vi "查找匹配累积剂量.vi"(8 "探头名称":string, 11 "累积剂量":T2(array[cluster])) -> (0 "匹配？":bool, 2 "匹配索引":i32, 3 "匹配的累积剂量":T1)   [LabVIEW 2017]
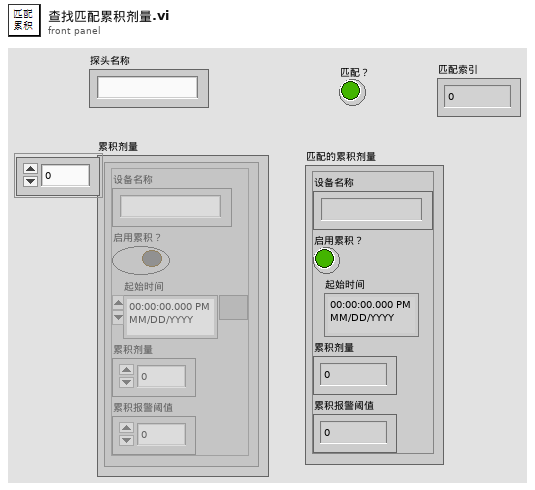
[diagram p1: front panel]
types:
  T1 = cluster{"设备名称":string, "启用累积？":bool, "起始时间":timestamp, "累积剂量":dbl, "累积报警阈值":dbl}
  T2 = cluster{"设备名称":string, "启用累积？":bool, "起始时间":timestamp, "累积剂量":dbl, "累积报警阈值":dbl}[]
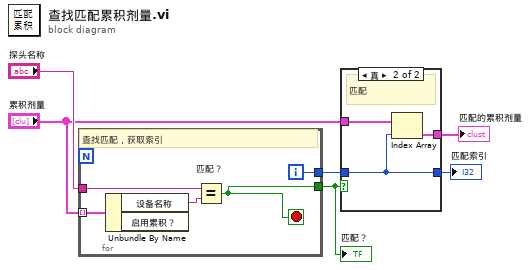
[diagram p0: block diagram]
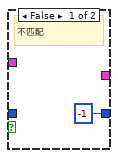
[diagram p2: hidden frame]
diagram:
  n1 = for {
    tunnel: "累积剂量" -> [w11] mode=indexing
    tunnel: "探头名称" -> [w9]
    tunnel: [w8] -> w4
    tunnel: [w7] -> w2
    i -> [w8]
    stop <- w7 stop-if-true
    # "查找匹配，获取索引"
    n2 = Unbundle By Name(w11) -> ("设备名称"=w10:string)  [unwired: 1 out]
    n3 = Equal? "匹配？"(x=w9, y=w10) -> (x = y?=w7:bool)
  }
  "匹配？" <- w2
  n4 = case shown="真" w2 {
    tunnel: "累积剂量" -> [_ w15]
    tunnel: w4 -> [_ w13]
    tunnel: [_ w14] -> w3
    tunnel: [-1 w13] -> w1
    frame False {
      # "不匹配"
    }
    frame True {
      # "匹配"
      n5 = Index Array(array=w15, index=w13) -> (element=w14:T1)
    }
  }
  "匹配的累积剂量" <- w3
  "匹配索引" <- w1
